vi "Get_Wavelength_Unit.vi"(8 "error in (no error)":errorcluster, 11 ".NET Reference in":refnum<k24>) -> (0 "error out":errorcluster, 2 "unit":i32(ring) items=["nm", "THz"], 3 "Reference out":refnum<k24>)   [LabVIEW 2017]
uses:
  LV_IL_Sample/DLL/InstrumentDLL.dll
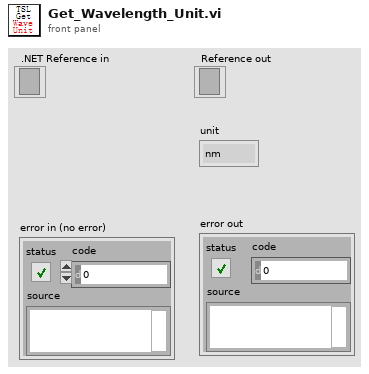
[diagram p1: front panel]
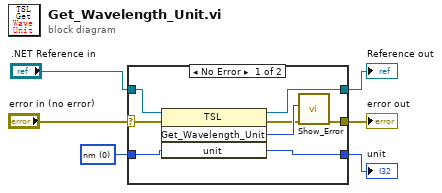
[diagram p0: block diagram]
diagram:
  w3 = 0 items=["nm", "THz"] ("unit")
  n1 = case shown="No Error" "error in (no error)" {
    selector: "error in (no error)" -> [w7 w16]
    tunnel: ".NET Reference in" -> [w14 w17]
    tunnel: [w13 w17] -> w5
    tunnel: [w8 w16] -> w4
    tunnel: w3 -> [w12 w15]
    tunnel: [w11 w15] -> w2
    frame No Error {
      n2 = invoke on="调用节点" class="TSL" method="Get_Wavelength_Unit"(reference=w14, error in=w7, "unit"=w12) -> (reference out=w13:refnum<k24>, error out=w9:errorcluster, "Get_Wavelength_Unit"=w10:i32, "unit"=w11:i32)  [unwired: 1 in]
      n3 = call "Show_Error.vi"("error in (no error)"=w9, "Error"=w10) -> ("error out"=w8:errorcluster)  [unwired: 9 in]
    }
    frame Error {
    }
  }
  "Reference out" <- w5
  "error out" <- w4
  "unit" <- w2
